vi "Set VI Refnum.vi"(8 "error in (no error)":errorcluster, 10 "VI Refnum":refnum<vi>, 11 "ESP Actor in":refnum<class "ESP Actor.lvclass">) -> (0 "error out":errorcluster, 3 "ESP Actor out":refnum<class "ESP Actor.lvclass">)   [LabVIEW 2020, in "ESP Actor.lvlib" / "ESP Actor.lvclass"]
uses:
  ESP Actor.lvclass
  ESP Actor.lvclass/ESP Actor.ctl
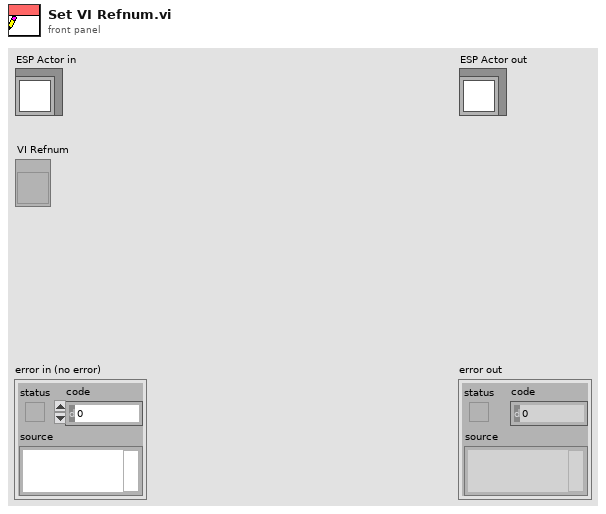
[diagram p1: front panel]
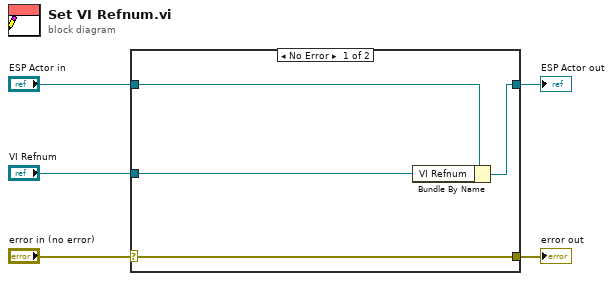
[diagram p0: block diagram]
diagram:
  n1 = case shown="No Error" "error in (no error)" {
    selector: "error in (no error)" -> [w9 w10]
    tunnel: [w9 w10] -> w4
    tunnel: [w7 w11] -> w2
    tunnel: "ESP Actor in" -> [w8 w11]
    tunnel: "VI Refnum" -> [w6 _]
    frame No Error {
      n2 = Bundle By Name(cluster=w8, "VI Refnum"=w6) -> (w7:refnum<class "ESP Actor.lvclass">)
    }
    frame Error {
    }
  }
  "error out" <- w4
  "ESP Actor out" <- w2
